vi "Autonomous Execution.vi"(8 "error in":errorcluster, 9 "Autonomous Queue":refnum<queue>, 11 "Queue Key":refnum<queue>) -> ()   [LabVIEW 2016]
uses:
  Robot Subsystems.ctl
  Drive/Drive Notifier.ctl
  Drive/Drive Control Type.ctl
  Climb/Climb Notifier.ctl
  Climb/Climb Control Type.ctl
  Intake/Intake Notifier.ctl
  Intake/Intake Control Type.ctl
  Rotation/Rotation Notifier.ctl
  Rotation/Rotation Control Type.ctl
  Queue Key Data.ctl
panel:
  out "error out":errorcluster
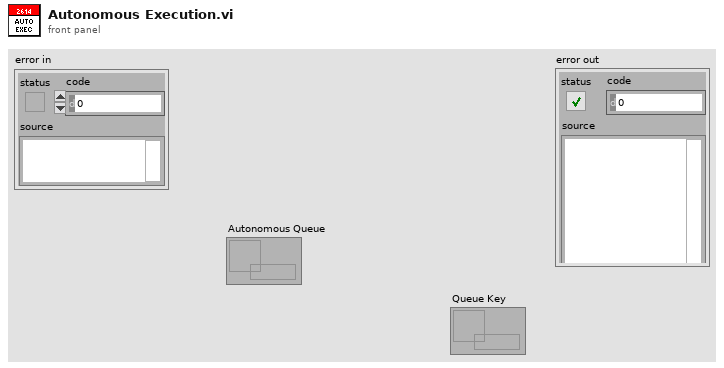
[diagram p1: front panel]
types:
  T1 = typedef "Queue Key Data.ctl" = cluster{"Operation Notifier":refnum<notifier>, "Subsystem":string, "Concurrent":bool}
  T2 = typedef "Robot Subsystems.ctl" = cluster{"Drive Notifier":T3, "Climb Notifier":T5, "Intake Notifier":T7, "Rotation Notifier":T9}
  T3 = typedef "Drive Notifier.ctl" = cluster{"Parameter 1":dbl, "Parameter 2":dbl, "Parameter 3":dbl, "Drive Control List":T4, "Parameter 4":dbl, "Gear Angle":dbl, "Parameter 6":dbl, "Parameter 7":dbl, "Parameter 8":dbl, "Parameter 9":dbl, "Robotcentric":bool, "Reset Gyro":bool, "Reset Wheels":bool, "Turn to Gear Left":bool, "Turn to Gear Center":bool, "Turn to Gear Right":bool, "Half Power":bool, "Drive Notifier":refnum<notifier>, "Step":i32}
  T4 = typedef "Drive Control Type.ctl" = enum16{"No Op", "Fieldcentric", "Robotcentric", "Reset Wheel Position", "Reset Gyro Value", "Turn to Angle", "Drive For Time"}
  T5 = typedef "Climb Notifier.ctl" = cluster{"Up":bool, "Down":bool, "Climb Control List":T6}
  T6 = typedef "Climb Control Type.ctl" = enum16{"No Op", "Up", "Down"}
  T7 = typedef "Intake Notifier.ctl" = cluster{"In":bool, "Out":bool, "Intake Control List":T8, "Parameter 1":dbl, "Parameter 2":dbl, "Intake Notifier":refnum<notifier>, "Step":i32}
  T8 = typedef "Intake Control Type.ctl" = enum16{"No Op", "In", "Out"}
  T9 = typedef "Rotation Notifier.ctl" = cluster{"Up":bool, "Down":bool, "Rotation Control List":T10, "Control Down":bool, "Manual":bool, "Parameter 1":dbl, "Parameter 2":dbl, "Rotation Notifier":refnum<notifier>, "Step":i32}
  T10 = typedef "Rotation Control Type.ctl" = enum16{"No Op", "Up", "Down", "Control Up", "Control Down"}
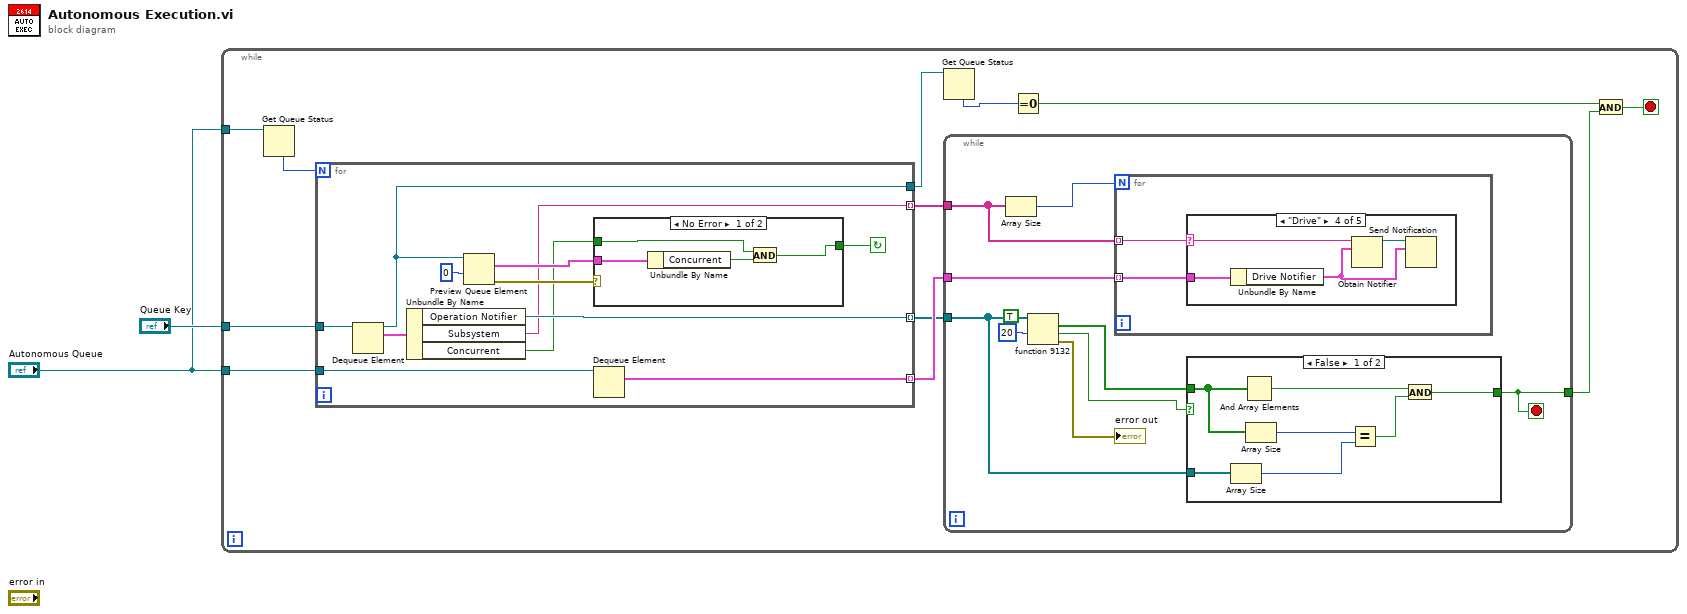
[diagram p0: block diagram]
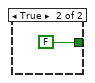
[diagram p2: hidden frame]
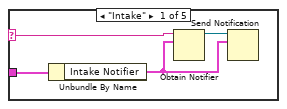
[diagram p3: hidden frame]
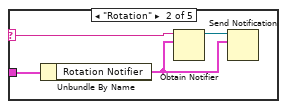
[diagram p4: hidden frame]
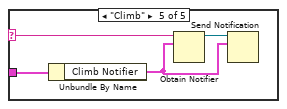
[diagram p6: hidden frame]
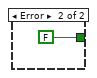
[diagram p7: hidden frame]
diagram:
  n1 = while {
    tunnel: "Queue Key" -> [w13]
    tunnel: "Autonomous Queue" -> [w14]
    tunnel: "Autonomous Queue" -> [w4]
    stop <- w6 stop-if-true
    n2 = Get Queue Status(queue=w4) -> (# elements in queue=w8:i32)  [unwired: 2 in, 7 out]
    n3 = for {
      N: w8 -> [_]
      tunnel: w14 -> [w56]
      tunnel: w13 -> [w62]
      tunnel: [w53] -> w9 mode=indexing
      tunnel: [w57] -> w3
      tunnel: [w52] -> w11 mode=indexing
      tunnel: [w55] -> w10 mode=indexing
      stop <- w58 continue-if-true
      n4 = Dequeue Element(queue=w62) -> (queue out=w57:refnum<queue>, element=w54:T1)  [unwired: 2 in, 2 out]
      n5 = Unbundle By Name(w54) -> ("Operation Notifier"=w53:refnum<notifier>, "Subsystem"=w52:string, "Concurrent"=w51:bool)
      n6 = Preview Queue Element(queue=w57, timeout in ms (-1)=0) -> (element=w61:T1, error out=w59:errorcluster)  [unwired: 1 in, 2 out]
      n7 = case shown="No Error" w59 {
        tunnel: w61 -> [w64 _]
        tunnel: [w66 FALSE] -> w58
        tunnel: w51 -> [w65 _]
        frame No Error {
          n8 = Unbundle By Name(w64) -> ("Concurrent"=w63:bool)
          n9 = And(x=w65, y=w63) -> (x .and. y?=w66:bool)
        }
        frame Error {
        }
      }
      n10 = Dequeue Element(queue=w56) -> (element=w55:T2)  [unwired: 2 in, 3 out]
    }
    n11 = Get Queue Status(queue=w3) -> (# elements in queue=w12:i32)  [unwired: 2 in, 7 out]
    n12 = while {
      tunnel: w11 -> [w19]
      tunnel: w10 -> [w24]
      tunnel: w9 -> [w16]
      tunnel: [w17] -> w5
      stop <- w17 stop-if-true
      n13 = Array Size(array=w19) -> (size(s)=w20:i32)
      n14 = fn#9132(0:w16, 1:TRUE ("ignore previous (F)"), 2:20 ("timeout in ms (-1)")) -> (9:w23:bool[], 10:w21:bool, 11:→"error out":errorcluster)  [unwired: 1 in, 1 out]
      n15 = for {
        N: w20 -> [_]
        tunnel: w19 -> [w34] mode=indexing
        tunnel: w24 -> [w33] mode=indexing
        n16 = case shown="\"Drive\"" w34 {
          selector: w34 -> [w36 w40 _ w46 w50]
          tunnel: w33 -> [w35 w39 _ w45 w49]
          frame "Intake" {
            n17 = Unbundle By Name(w35) -> ("Intake Notifier"=w37:T7)
            n18 = Obtain Notifier(name (unnamed)=w36, notification data type=w37) -> (notifier out=w38:refnum<notifier>)  [unwired: 2 in, 2 out]
            n19 = Send Notification(notification=w37, notifier=w38) -> ()  [unwired: 1 in, 2 out]
          }
          frame "Rotation" {
            n20 = Unbundle By Name(w39) -> ("Rotation Notifier"=w41:T9)
            n21 = Obtain Notifier(name (unnamed)=w40, notification data type=w41) -> (notifier out=w42:refnum<notifier>)  [unwired: 2 in, 2 out]
            n22 = Send Notification(notification=w41, notifier=w42) -> ()  [unwired: 1 in, 2 out]
          }
          frame "No Op", Default {
          }
          frame "Drive" {
            n23 = Unbundle By Name(w45) -> ("Drive Notifier"=w43:T3)
            n24 = Obtain Notifier(name (unnamed)=w46, notification data type=w43) -> (notifier out=w44:refnum<notifier>)  [unwired: 2 in, 2 out]
            n25 = Send Notification(notification=w43, notifier=w44) -> ()  [unwired: 1 in, 2 out]
          }
          frame "Climb" {
            n26 = Unbundle By Name(w49) -> ("Climb Notifier"=w47:T5)
            n27 = Obtain Notifier(name (unnamed)=w50, notification data type=w47) -> (notifier out=w48:refnum<notifier>)  [unwired: 2 in, 2 out]
            n28 = Send Notification(notification=w47, notifier=w48) -> ()  [unwired: 1 in, 2 out]
          }
        }
      }
      n29 = case shown="False" w21 {
        tunnel: [w30 FALSE] -> w17
        tunnel: w23 -> [w29 _]
        tunnel: w16 -> [w28 _]
        frame False {
          n30 = Array Size(array=w28) -> (size(s)=w26:i32)
          n31 = And Array Elements(Boolean array=w29) -> (logical AND=w31:bool)
          n32 = Array Size(array=w29) -> (size(s)=w27:i32)
          n33 = Equal?(x=w27, y=w26) -> (x = y?=w25:bool)
          n34 = And(x=w31, y=w25) -> (x .and. y?=w30:bool)
        }
        frame True {
        }
      }
    }
    n35 = Equal To 0?(x=w12) -> (x = 0?=w7:bool)
    n36 = And(x=w7, y=w5) -> (x .and. y?=w6:bool)
  }
